vi "Write Registration Types.vi"(10 "Requested Registration Types":T1[](array[typedef]), 11 "IEventHandler In":refnum<class "IEventHandler.lvclass">) -> (0 "error out":errorcluster, 3 "IEventHandler Out":refnum<class "IEventHandler.lvclass">)   [LabVIEW 2017, in "ActorEvents.lvlib" / "IEventHandler.lvclass"]
uses:
  IEventHandler.lvclass
  <vilib>/event_ctls.llb/lveventtype.ctl
  IEventHandler.lvclass/IEventHandler.ctl
  <vilib>/Utility/error.llb/Error Cluster From Error Code.vi
  <vilib>/ErrorRing/Error Ring.xnode
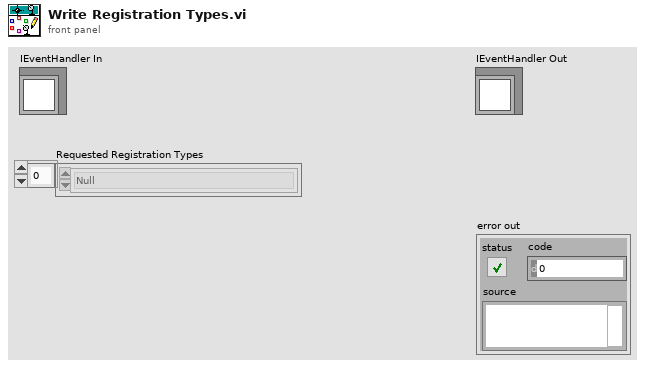
[diagram p1: front panel]
types:
  T1 = typedef "lveventtype.ctl" = enum32{"Null", "Timeout", "Annotation Menu Selection", "Annotation Menu Selection?", "App Instance Close", "App Instance Close?", "Autoscale Range Change", "Bookmark Info Change", "Cell Edit", "Cell Edit?", "Cursor Grab", "Cursor Grab?", "Cursor Menu Selection", "Cursor Menu Selection?", "Cursor Move", "Cursor Release", "Data Change", "Direction Change", "Display State Change", "Drag Ended", "Drag Enter", "Drag Leave", "Drag Over", "Drag Source Update", "Drag Starting", "Drag Starting?", "Drop", "Exec State Change", "Key Down", "Key Down?", "Key Repeat", "Key Repeat?", "Key Up", "Listbox Double Click", "Menu Activation?", "Menu Selection (App)", "Menu Selection? (App)", "Menu Selection (User)", "Mouse Down", "Mouse Down?", "Mouse Enter", "Mouse Leave", "Mouse Move", "Mouse Up", "Mouse Wheel", "NI Security User Change (App)", "Pane Size", "Panel Close", "Panel Close?", "Panel Resize", "Plot Attribute Change", "Scale Range Change", "Shortcut Menu Activation?", "Shortcut Menu Selection (App)", "Shortcut Menu Selection? (App)", "Shortcut Menu Selection (User)", "Tree Double Click", "Tree Drag", "Tree Drag?", "Tree Drop", "Tree Drop?", "Tree Item Close", "Tree Item Close?", "Tree Item Open", "Tree Item Open?", "User Event", "Value Change"}
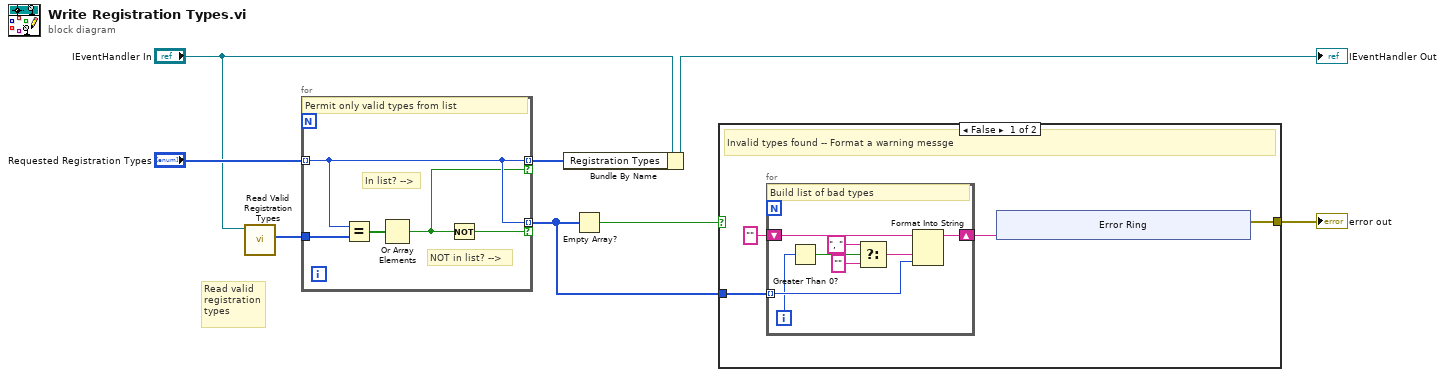
[diagram p0: block diagram]
diagram:
  # "Read valid\nregistration\ntypes"
  n1 = call-dynamic "Read Valid Registration Types.vi"("EventHandler Type"="IEventHandler In") -> ("Valid Registration Types"=w6:T1[])  [unwired: 10 in]
  n2 = for {
    tunnel: "Requested Registration Types" -> [w11] mode=indexing
    tunnel: w6 -> [w13]
    tunnel: [w11] -> w4 mode=indexing if=w9
    tunnel: [w11] -> w8 mode=indexing if=w10
    # "NOT in list? -->"
    # "In list? -->"
    # "Permit only valid types from list"
    n3 = Equal?(x=w11, y=w13) -> (x = y?=w12:bool[])
    n4 = Or Array Elements(Boolean array=w12) -> (logical OR=w9:bool)
    n5 = Not(x=w9) -> (.not. x?=w10:bool)
  }
  n6 = Bundle By Name(cluster="IEventHandler In", "Registration Types"=w4) -> (→"IEventHandler Out":refnum<class "IEventHandler.lvclass">)
  n7 = Empty Array?(array=w8) -> (empty?=w1:bool)
  n8 = case shown="False" w1 {
    tunnel: w8 -> [w16 _]
    tunnel: [w14 _] -> w2
    frame False {
      # "Invalid types found -- Format a warning messge"
      n9 = for {
        tunnel: w16 -> [w23] mode=indexing
        shift-right: [w25] -> w15
        shift-left: "" -> [w24]
        i -> [w22]
        # "Build list of bad types"
        n10 = Greater Than 0?(x=w22) -> (x > 0?=w21:bool)
        n11 = Select(t=", ", s=w21, f="") -> (s? t:f=w18:string)
        n12 = Format Into String(initial string=w24, w18, w23) -> (resulting string=w25:string)  [unwired: 2 in, 1 out]
      }
      n13 = xnode "Error Ring"("parameter 0"=w15) -> ("error out"=w14:errorcluster)
    }
    frame True {
      # "No invalid types found -- No warning"
    }
  }
  "error out" <- w2
